vi "EdgeDetection_Setting_UI.vi"(6 "Analysis_Setting IN":T2={"PreProcess"=enum."*Algorithm*", "Parameter"=""}, 8 "error in (no error)":errorcluster, 9 "ProjectName":string, 10 "ROI List IN":refnum<vi>, 11 "Vision_Image":T8(plugin-control)) -> (0 "error out":errorcluster, 1 "Cancel?":bool, 3 "Analysis_Setting":T2={"PreProcess"=enum."*Algorithm*", "Parameter"=""})   [LabVIEW 2019]
uses:
  <vilib>/userdefined/High Color/IMAQdx.ctl
  <vilib>/vision/NI_Vision_Development_Module.lvlib
  Controls/_UI Command Cluster/Edge Detection_UI Command Cluster.ctl
  Controls/Edge Detection/Analysis_Edge Detection_Parameter.ctl
  Controls/Analysis_Type.ctl
  Controls/Analysis_Setting.ctl
  Controls/V_Analysis_Type.ctl
  <vilib>/vision/Measure.llb/Edge New.ctl
  Ctrl/VisionProcessName.ctl
panel:
  in  "Snap?":bool
  in  "ROI Descriptor":T1
  out "Numeric":i32
  in  "Done":bool
  in  "Cancel":bool
  in  "EdgeDetectionTab":T4(tab)
  in  "Number of Matches Requested":i32=1 min=1 max=9999
  in  "Process":T5(ring)=enum."Get All Edges"
  in  "Edge Options":T6={"Edge Polarity"=enum."All Edges", "Kernel Size"=3, "Width"=5, "Minimum Edge Strength"=10.0, "Interpolation Type"=enum."Bilinear", "Data Processing Method"=enum."Average"} {"Width" min=1 step=2; "Kernel Size" min=3 step=2; "Minimum Edge Strength" min=0.0 max=255.0 format="%.2g"}
  out "Number of Edges Detected":i32
  out "Edge Information":T7[](array[typedef]) {"Distance (Real-World)" format="%.2f"; "Location (Real-World)"."Y" format="%.2g"; "Location (Real-World)"."X" format="%.2f"; "Noise" format="%.2f"; "Location (Pixel)"."Y" format="%.2g"; "Location (Pixel)"."X" format="%.2f"; "Strength" format="%.2f"; "Distance (Pixel)" format="%.2f"}
  in  "Edge Detection_UI Command":T9(ring)
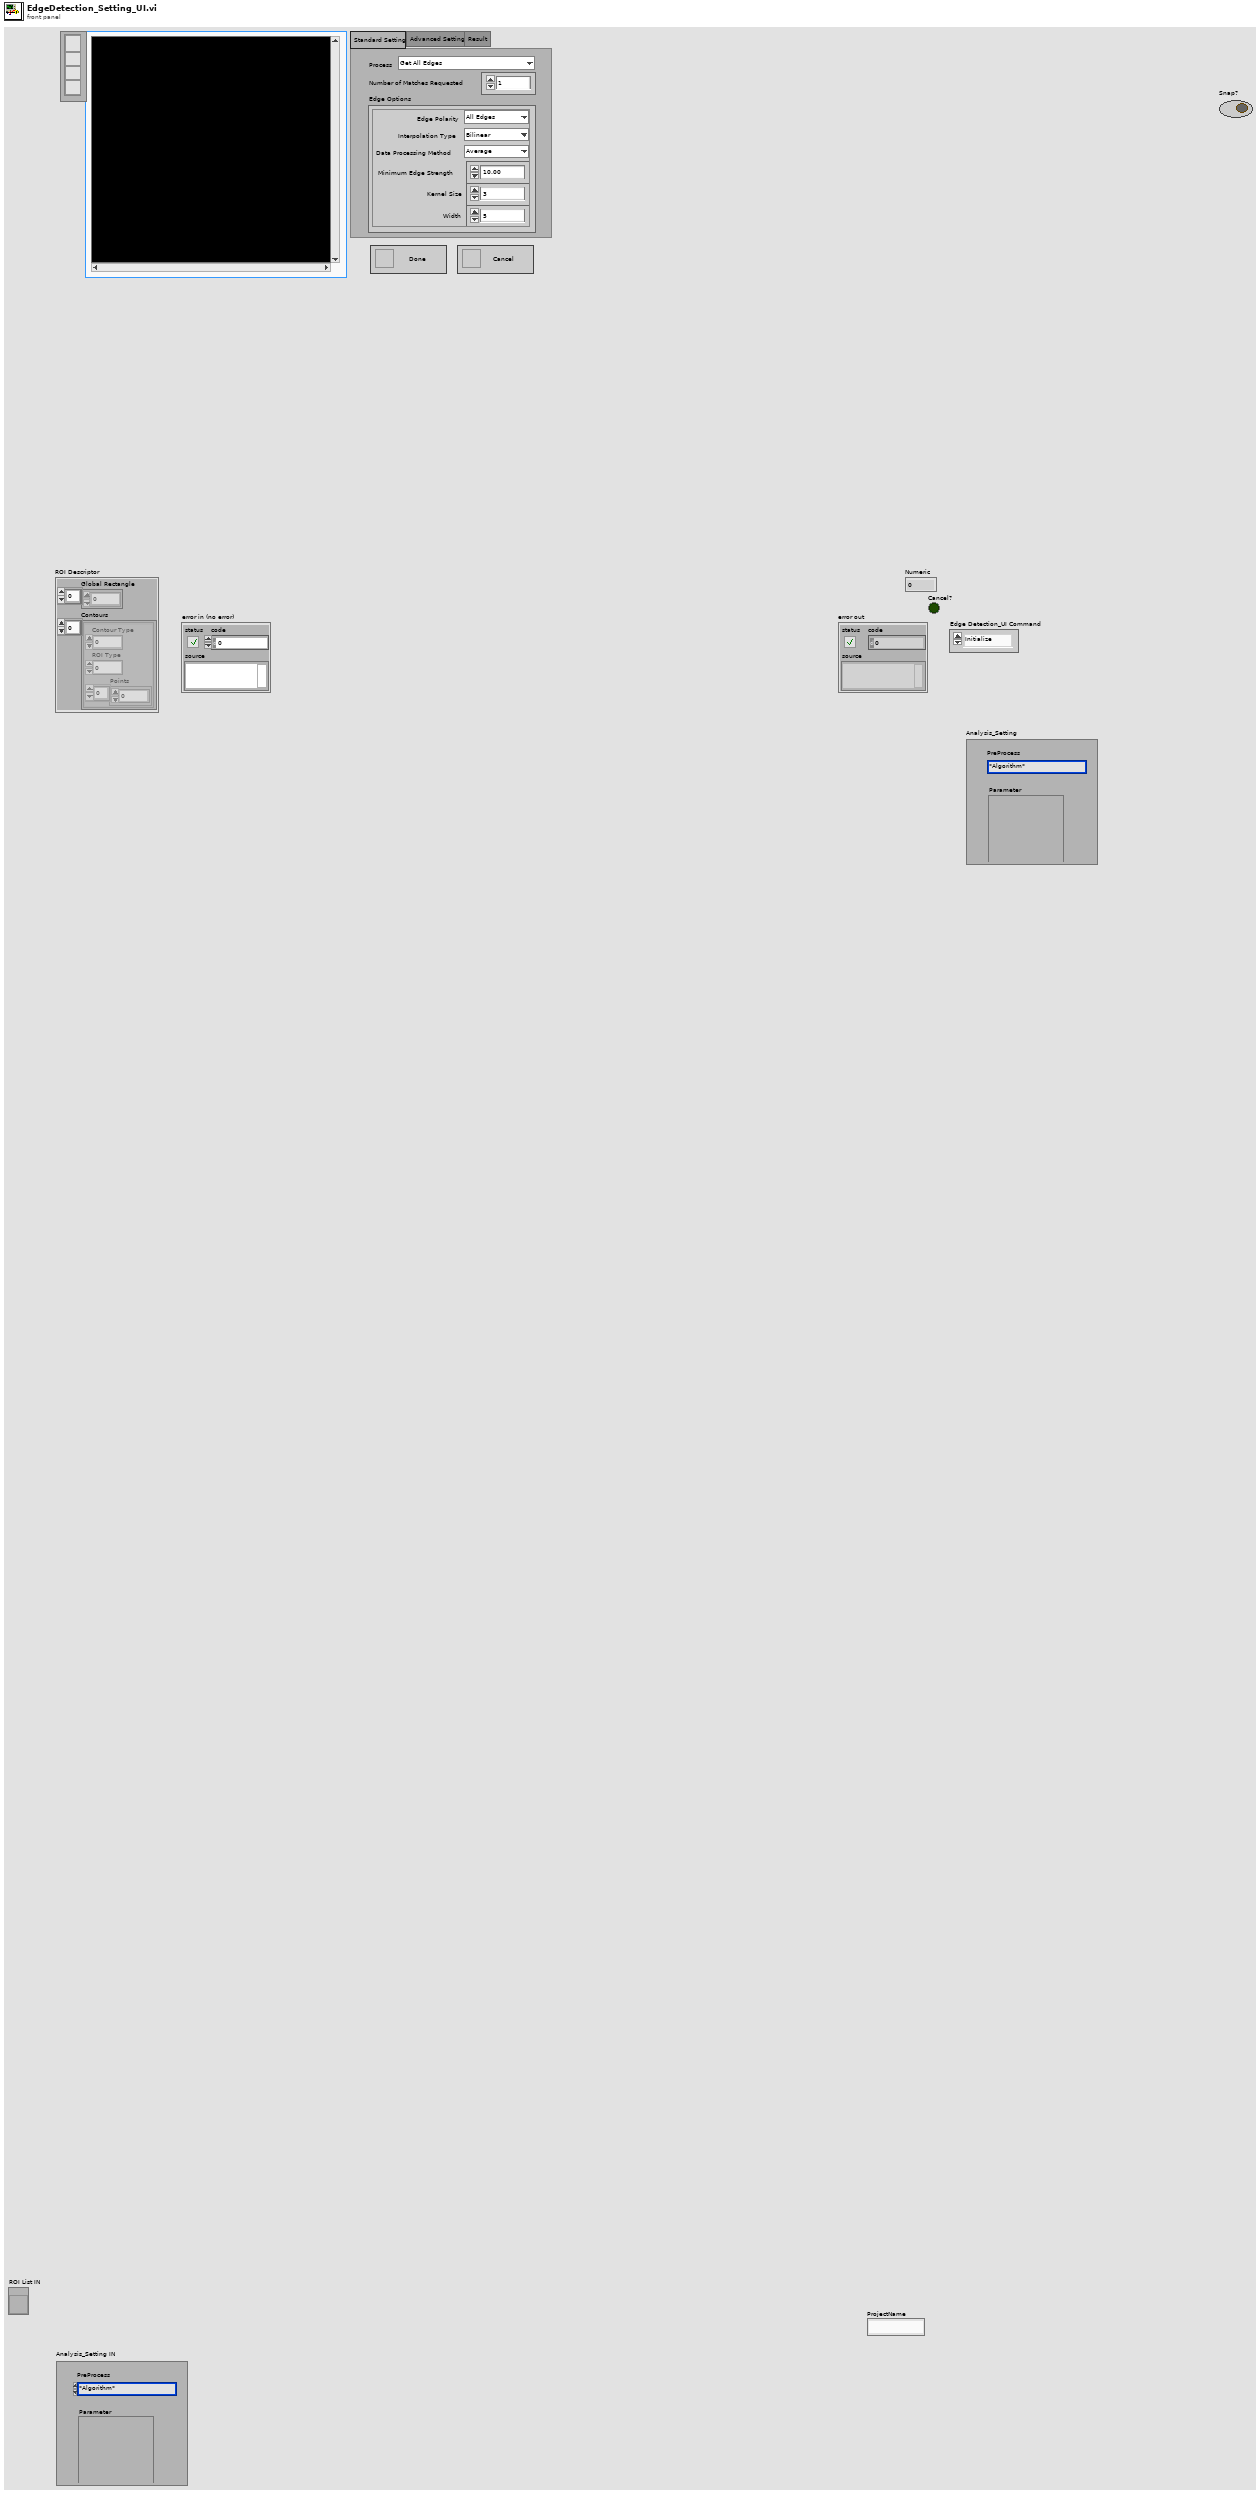
[diagram p1: front panel]
types:
  T1 = cluster{"Global Rectangle":i32[], "Contours":cluster{"Contour Type":u32, "ROI Type":u32, "Points":i32[]}[]}
  T2 = typedef "Analysis_Setting.ctl" = cluster{"PreProcess":T3, "Parameter":string}
  T3 = typedef "VisionProcessName.ctl" = enum16{"*CamParameter*", "CamAttributes", "*Preprocess*", "CG_Brightness", "C_Plane Extraction", "C_Threshold", "G_Lookup Table", "G_Threshold", "B_Image Inversion", "*Algorithm*", "CG_Histogram", "C_Color Matching", "C_Color Pattern Matching", "G_PatternMatch", "CG_Find Straight Edge", "CG_Adv. Find Straight Edge", "CG_Find Circular Edge", "G_Max Clamp", "G_Clamp (Rake)", "G_Pattern Matching"}
  T4 = enum32{"Standard Setting", "Advanced Setting", "Result"}
  T5 = enum16{"Get First Edge", "Get First + Last Edge", "Get All Edges", "Get Best Edge"}
  T6 = cluster{"Edge Polarity":enum16{"All Edges", "Rising Edges", "Falling Edges"}, "Kernel Size":u32, "Width":u32, "Minimum Edge Strength":dbl, "Interpolation Type":enum16{"Zero Order", "Bilinear", "Bilinear Fixed"}, "Data Processing Method":enum16{"Average", "Median"}}
  T7 = typedef "Edge New.ctl" = cluster{"Location (Pixel)":cluster{"X":sgl, "Y":sgl}, "Location (Real-World)":cluster{"X":sgl, "Y":sgl}, "Distance (Pixel)":dbl, "Distance (Real-World)":dbl, "Strength":dbl, "Noise":dbl, "Rising?":bool}
  T8 = typedef "IMAQ Image.ctl" = refnum<image>
  T9 = enum16{"Initialize", "Done", "Run Algorithm", "Cancel"}
  T10 = typedef "Analysis_Edge Detection_Parameter.ctl" = cluster{"Edge Options":cluster{"Edge Polarity":u16, "Kernel Size":u32, "Width":u32, "Minimum Edge Strength":dbl, "Interpolation Type":u16, "Data Processing Method":u16}, "Process":u16, "Number of Matches Requested":i32, "ROI Descriptor":cluster{"Global Rectangle":i32[], "Contours":cluster{"Contour Type":u32, "ROI Type":u32, "Points":i32[]}[]}}
  T11 = typedef "Edge Detection_UI Command Cluster.ctl" = cluster{"Edge Detection_UI Command":enum16{"Initialize", "Done", "Run Algorithm", "Cancel"}, "Edge Options":cluster{"Edge Polarity":u16, "Kernel Size":u32, "Width":u32, "Minimum Edge Strength":dbl, "Interpolation Type":u16, "Data Processing Method":u16}, "Process":u16, "Number of Matches Requested":i32, "ROI Descriptor":cluster{"Global Rectangle":i32[], "Contours":cluster{"Contour Type":u32, "ROI Type":u32, "Points":i32[]}[]}, "Snap Simulation Mouse Down":bool}
  T12 = typedef "IMAQ Line" = cluster{"Start X":i32, "Start Y":i32, "End X":i32, "End Y":i32}
  T13 = typedef "IMAQdx.ctl" = refnum<k21>
  T14 = cluster{"Contour Type":u32, "ROI Type":u32, "Points":i32[]}
  T15 = cluster{"Edge Polarity":u16, "Kernel Size":u32, "Width":u32, "Minimum Edge Strength":dbl, "Interpolation Type":u16, "Data Processing Method":u16}
  T16 = typedef "Image Type" = u32
  T17 = typedef "Analysis_Type.ctl" = u16
  T18 = typedef "ROI Descriptor" = cluster{"Global Rectangle":i32[], "Contours":cluster{"ID":enum32{"External", "Internal"}, "Type":u32, "Coordinates":i32[]}[]}
  T19 = typedef "Analysis_Setting.ctl" = cluster{"PreProcess":T20, "Parameter":string}
  T20 = typedef "V_Analysis_Type.ctl" = enum16{"None", "C_Color Pattern Matching", "G_PatternMatching", "G_ShapeDectect", "G_GeometricMatch", "B_Area Check"}
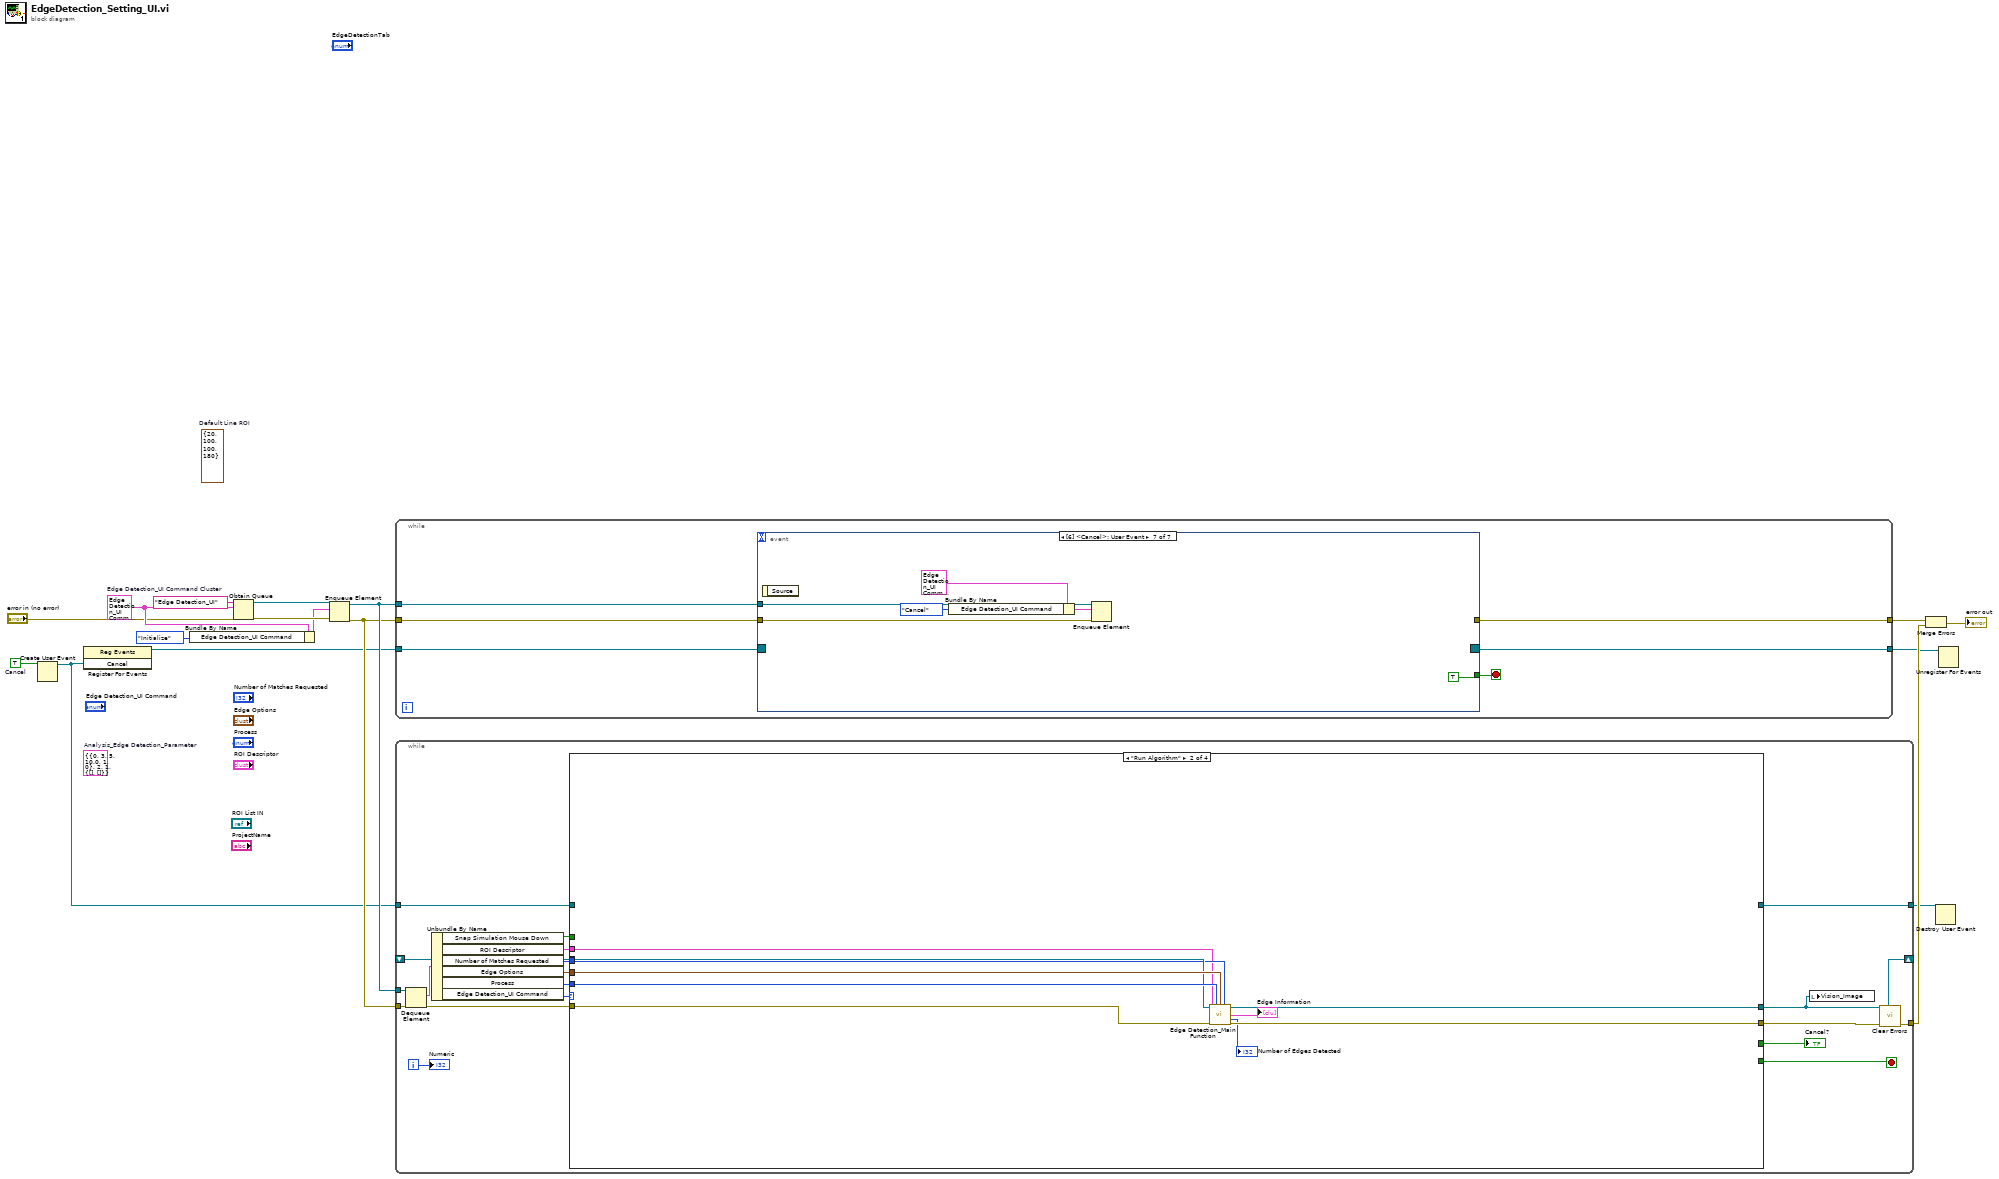
[diagram p0: block diagram]
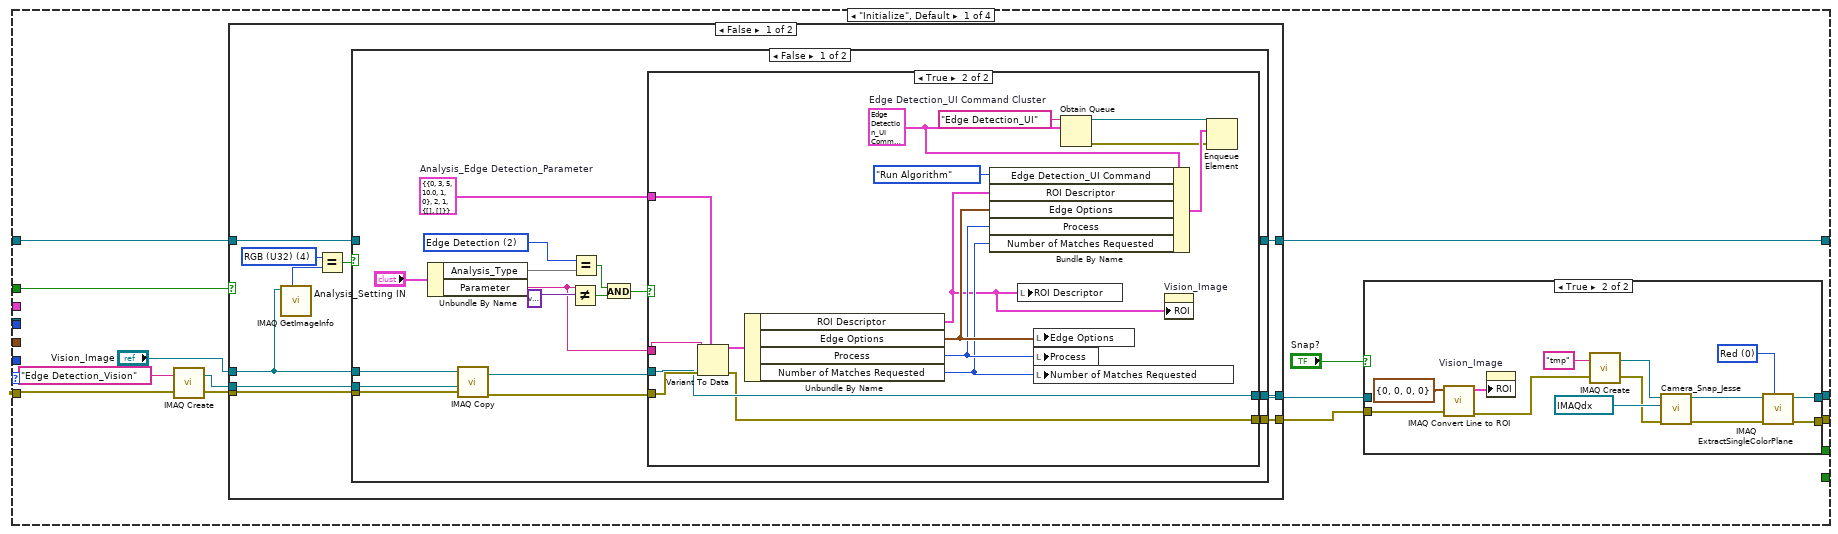
[diagram p2: hidden frame]
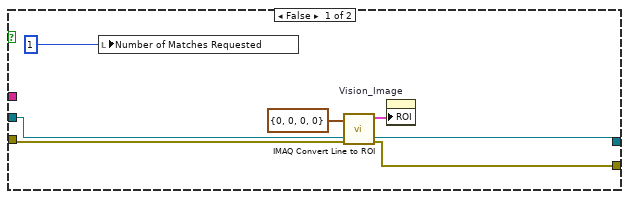
[diagram p4: hidden frame]
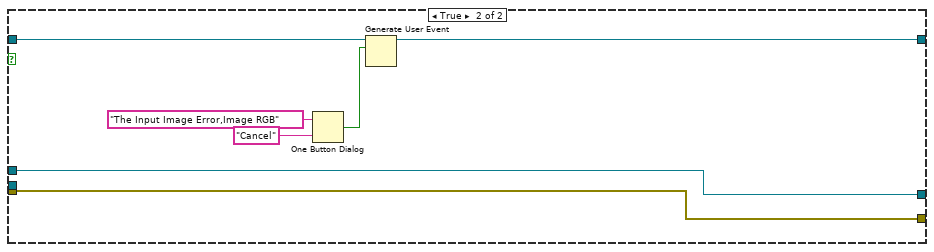
[diagram p5: hidden frame]
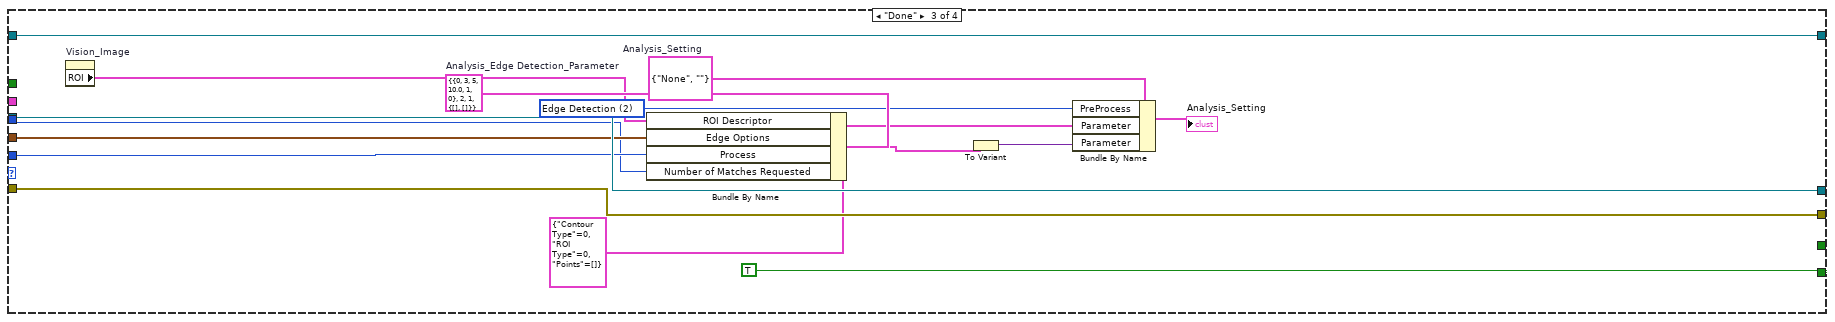
[diagram p7: hidden frame]
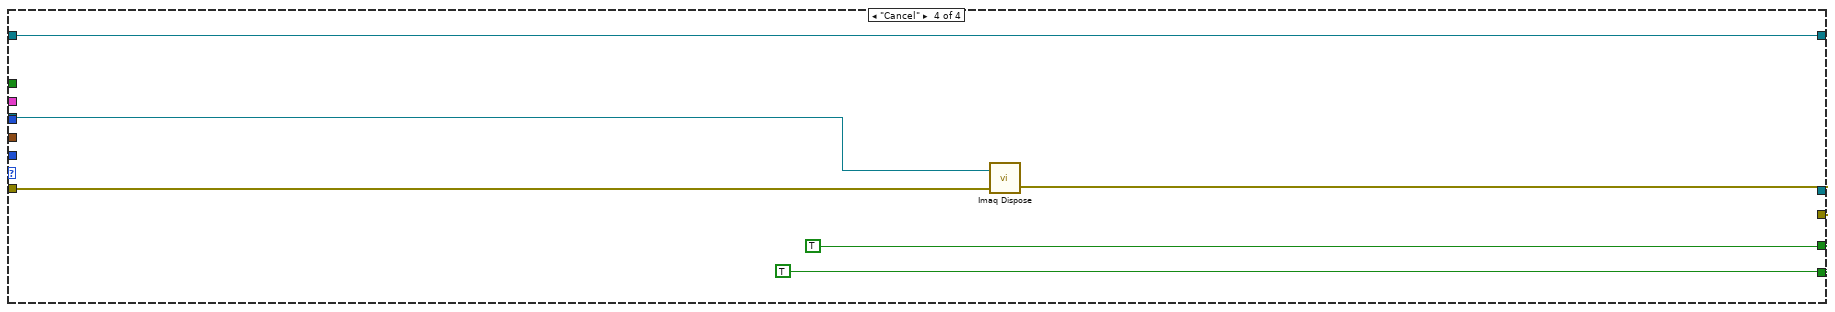
[diagram p8: hidden frame]
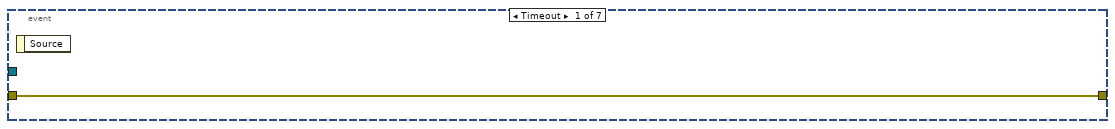
[diagram p9: hidden frame]
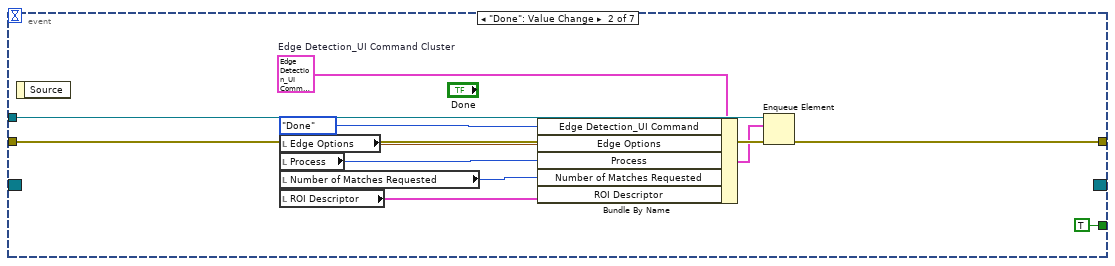
[diagram p10: hidden frame]
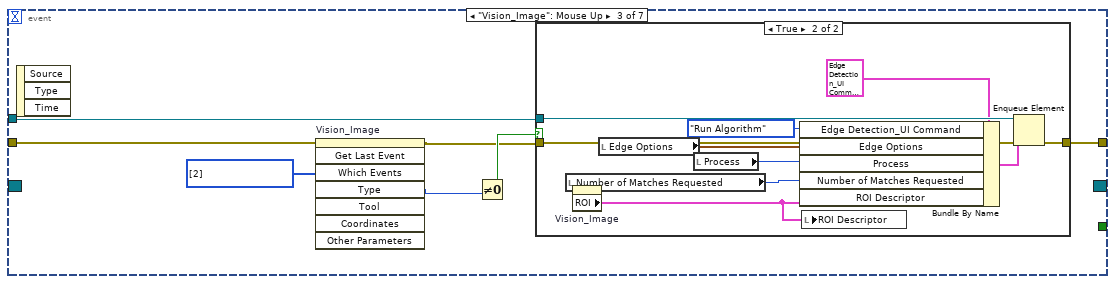
[diagram p11: hidden frame]
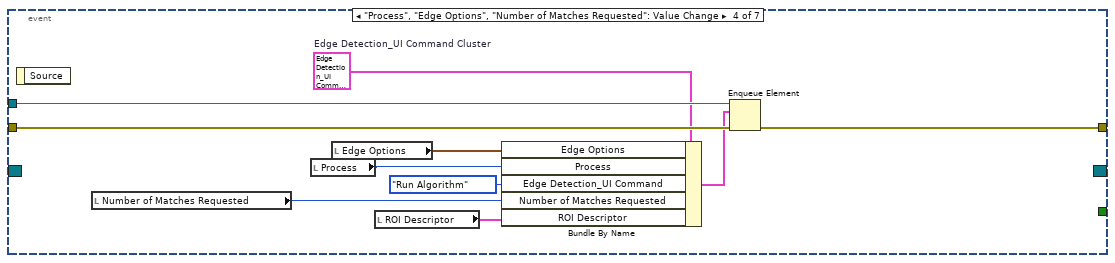
[diagram p13: hidden frame]
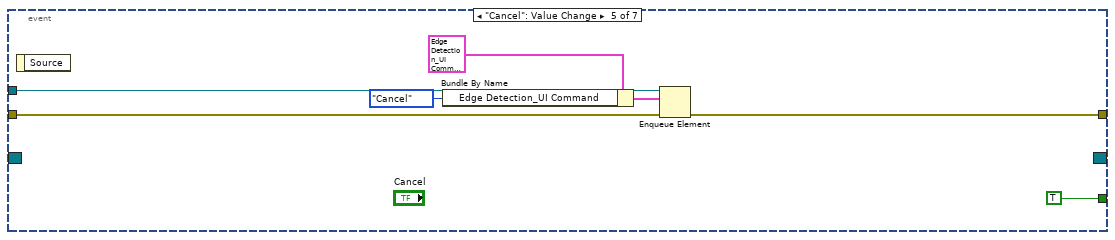
[diagram p14: hidden frame]
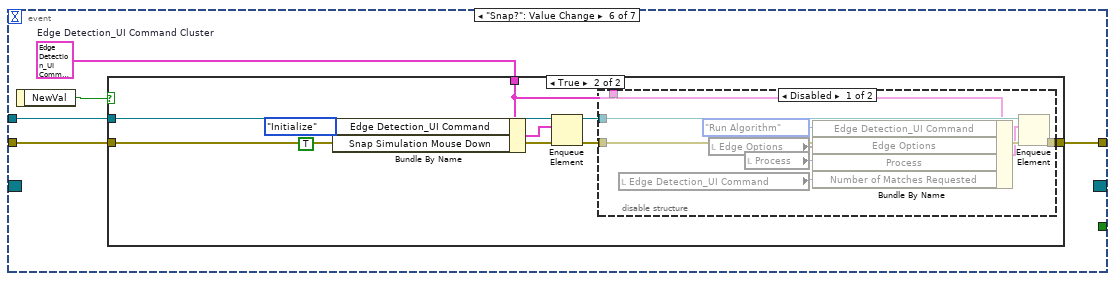
[diagram p15: hidden frame]
diagram:
  (unwired) T10 {"Edge Options"={"Edge Polarity"=0, "Kernel Size"=3, "Width"=5, "Minimum Edge Strength"=10.0, "Interpolation Type"=1, "Data Processing Method"=0}, "Process"=2, "Number of Matches Requested"=1, "ROI Descriptor"={"Global Rectangle"=[], "Contours"=[]}}  # Analysis_Edge Detection_Parameter
  w5 = TRUE  # Cancel
  w10 = T11 {"Edge Detection_UI Command"=enum."Initialize", "Edge Options"={"Edge Polarity"=0, "Kernel Size"=3, "Width"=5, "Minimum Edge Strength"=10.0, "Interpolation Type"=1, "Data Processing Method"=0}, "Process"=2, "Number of Matches Requested"=1, "ROI Descriptor"={"Global Rectangle"=[], "Contours"=[]}, "Snap Simulation Mouse Down"=FALSE}  # Edge Detection_UI Command Cluster
  (unwired) T12 {"Start X"=20, "Start Y"=100, "End X"=100, "End Y"=180}  # Default Line ROI
  n1 = Create User Event(user event datatype=w5) -> (user event=w3:refnum<user-event>)  [unwired: 1 in, 1 out]
  n2 = register-events(w3) -> (reference out=w4:refnum<event-registration>)  [unwired: 2 in, 1 out]
  n3 = Bundle By Name(cluster=w10, "Edge Detection_UI Command"=T9."Initialize") -> (w9:T11)
  n4 = Obtain Queue(name (unnamed)="Edge Detection_UI", element data type=w10, error in (no error)="error in (no error)") -> (queue out=w17:refnum<queue>, error out=w16:errorcluster)  [unwired: 2 in, 1 out]
  n5 = Enqueue Element(queue=w17, element=w9, error in (no error)=w16) -> (queue out=w14:refnum<queue>, error out=w13:errorcluster)  [unwired: 1 in, 1 out]
  n6 = while {
    tunnel: w14 -> [w36]
    tunnel: w13 -> [w35]
    shift-right: [w26] -> _
    shift-left: _ -> [w29]
    tunnel: [w19] -> w11
    tunnel: w3 -> [w21]
    tunnel: [w20] -> w1
    i -> [w27]
    stop <- w30 stop-if-true
    n7 = Dequeue Element(queue=w36, error in (no error)=w35) -> (element=w32:T11, error out=w33:errorcluster)  [unwired: 1 in, 2 out]
    n8 = Unbundle By Name(w32) -> ("Snap Simulation Mouse Down"=w22:bool, "ROI Descriptor"=w23:T1, "Number of Matches Requested"=w24:i32, "Edge Options"=w31:T15, "Process"=w28:u16, "Edge Detection_UI Command"=w34:T9)
    n9 = case shown="\"Run Algorithm\"" w34 {
      tunnel: w33 -> [w48 w131 w145 w150]
      tunnel: [w40 w128 w145 w149] -> w18
      tunnel: w31 -> [_ w130 w143 _]
      tunnel: [_ _ TRUE TRUE] -> w30
      tunnel: [w41 w127 w144 _] -> w26
      tunnel: w29 -> [_ w126 w144 w151]
      tunnel: w28 -> [_ w129 w142 _]
      tunnel: [_ _ _ TRUE] -> w25
      tunnel: w24 -> [_ w125 w134 _]
      tunnel: w23 -> [_ w123 _ _]
      tunnel: w22 -> [w47 _ _ _]
      tunnel: w21 -> [w38 _ w132 w147]
      tunnel: [w37 _ w132 w147] -> w20
      frame "Initialize", Default {
        n10 = call "IMAQ Create"("Image Name"="Edge Detection_Vision", "error in (no error)"=w48) -> ("New Image"=w46:T8, "error out"=w45:errorcluster)  [unwired: 3 in]
        n11 = case shown="False" w47 {
          tunnel: [w74 w120] -> w42
          tunnel: [w73 w121] -> w43
          tunnel: w45 -> [w72 w120]
          tunnel: "Vision_Image" -> [w70 _]
          tunnel: w46 -> [w71 w121]
          tunnel: w38 -> [w66 _]
          tunnel: [w65 _] -> w37
          frame False {
            w68 = T16 4 items=["Grayscale (U8)", "Grayscale (I16)", "Grayscale (SGL)", "Complex (CSG)", "RGB (U32)", "HSL (U32)", "RGB (U64)", "Grayscale (U16)"] ("x")
            n12 = call "IMAQ GetImageInfo"("Image"=w70) -> ("Image Type"=w69:T16)  [unwired: 3 in, 7 out]
            n13 = Equal?(x=w68, y=w69) -> (x = y?=w67:bool)
            n14 = case shown="False" w67 {
              tunnel: [w90 w117] -> w74
              tunnel: [w89 w114] -> w73
              tunnel: w72 -> [w79 w117]
              tunnel: w71 -> [w76 _]
              tunnel: w70 -> [w75 w114]
              tunnel: w66 -> [_ w115]
              tunnel: [_ w113] -> w65
              frame False {
                w80 = T10 {"Edge Options"={"Edge Polarity"=0, "Kernel Size"=3, "Width"=5, "Minimum Edge Strength"=10.0, "Interpolation Type"=1, "Data Processing Method"=0}, "Process"=2, "Number of Matches Requested"=1, "ROI Descriptor"={"Global Rectangle"=[], "Contours"=[]}}  # Analysis_Edge Detection_Parameter
                w86 = T17 2 items=["None", "PatternMatch", "Edge Detection", "Barcode 1D", "Barcode 2D", "Clamp", "Clamp MAX", "Particle", "Histogram", "Straight Edge", "Circle", "Shape Detect", "OCR", "Contour", "ColorMatch"] ("x")
                n15 = Unbundle By Name("Analysis_Setting IN") -> ("Analysis_Type"=w85, "Parameter"=w82:string)
                n16 = call "IMAQ Copy"("error in (no error)"=w79, "Image Dst"=w76, "Image Src"=w75) -> ("error out"=w77:errorcluster, "Image Dst Out"=w78:T8)  [unwired: 3 in]
                n17 = Not Equal?(x=w82, y=variant) -> (x != y?=w87:bool)
                n18 = Equal?(x=w86, y=w85) -> (x = y?=w88:bool)
                n19 = And(x=w88, y=w87) -> (x .and. y?=w83:bool)
                n20 = case shown="True" w83 {
                  tunnel: w77 -> [w92 w110]
                  tunnel: [w91 w98] -> w90
                  tunnel: [w95 w99] -> w89
                  tunnel: w82 -> [_ w112]
                  tunnel: w78 -> [w95 w99]
                  tunnel: w80 -> [_ w103]
                  frame False {
                    n21 = local write "Number of Matches Requested"(1 ("Number of Matches Requested")) -> ()
                    n22 = call "IMAQ Convert Line to ROI"("error in (no error)"=w92, "Line"=T12 {"Start X"=0, "Start Y"=0, "End X"=0, "End Y"=0}) -> ("error out"=w91:errorcluster, "ROI Descriptor"=w93:T18)  [unwired: 7 in]
                    n23 = property on="Vision_Image" class="ImageControl"("ROI"=w93) -> ()  [unwired: 2 in, 2 out]
                  }
                  frame True {
                    w108 = T11 {"Edge Detection_UI Command"=enum."Initialize", "Edge Options"={"Edge Polarity"=0, "Kernel Size"=3, "Width"=5, "Minimum Edge Strength"=10.0, "Interpolation Type"=1, "Data Processing Method"=0}, "Process"=2, "Number of Matches Requested"=1, "ROI Descriptor"={"Global Rectangle"=[], "Contours"=[]}, "Snap Simulation Mouse Down"=FALSE}  # Edge Detection_UI Command Cluster
                    n24 = Variant To Data(error in=w110, type=w103, Variant=w112) -> (data=w111:T10, error out=w98:errorcluster)
                    n25 = Unbundle By Name(w111) -> ("ROI Descriptor"=w97:T1, "Edge Options"=w102:T15, "Process"=w101:u16, "Number of Matches Requested"=w100:i32)
                    n26 = Bundle By Name(cluster=w108, "Edge Detection_UI Command"=T9."Run Algorithm", "ROI Descriptor"=w97, "Edge Options"=w102, "Process"=w101, "Number of Matches Requested"=w100) -> (w109:T11)
                    n27 = local write "ROI Descriptor"(w97) -> ()
                    n28 = local write "Edge Options"(w102) -> ()
                    n29 = local write "Process"(w101) -> ()
                    n30 = local write "Number of Matches Requested"(w100) -> ()
                    n31 = Obtain Queue(name (unnamed)="Edge Detection_UI", element data type=w108) -> (queue out=w105:refnum<queue>, error out=w106:errorcluster)  [unwired: 3 in, 1 out]
                    n32 = property on="Vision_Image" class="ImageControl"("ROI"=w97) -> ()  [unwired: 2 in, 2 out]
                    n33 = Enqueue Element(queue=w105, element=w109, error in (no error)=w106) -> ()  [unwired: 1 in, 3 out]
                  }
                }
              }
              frame True {
                n34 = One Button Dialog(message="The Input Image Error,Image RGB", button name ("OK")="Cancel") -> (true=w116:bool)
                n35 = Generate User Event(user event=w115, event data cluster=w116) -> (user event out=w113:refnum<user-event>)  [unwired: 2 in, 1 out]
              }
            }
          }
          frame True {
          }
        }
        n36 = case shown="True" "Snap?" {
          tunnel: [w51 w57] -> w40
          tunnel: [w50 w56] -> w41
          tunnel: w42 -> [w51 w53]
          tunnel: w43 -> [w50 _]
          frame False {
          }
          frame True {
            w60 = 0 items=["Red", "Green", "Blue", "Hue", "Saturation", "Luminance", "Value", "Intensity"] ("Color Plane")
            n37 = call "IMAQ Convert Line to ROI"("error in (no error)"=w53, "Line"=T12 {"Start X"=0, "Start Y"=0, "End X"=0, "End Y"=0}) -> ("error out"=w52:errorcluster, "ROI Descriptor"=w54:T18)  [unwired: 7 in]
            n38 = property on="Vision_Image" class="ImageControl"("ROI"=w54) -> ()  [unwired: 2 in, 2 out]
            n39 = call "IMAQ Create"("Image Name"="tmp", "error in (no error)"=w52) -> ("New Image"=w62:T8, "error out"=w59:errorcluster)  [unwired: 3 in]
            n40 = call "Camera_Snap_Jesse.vi"("error in (no error)"=w59, "Camera Session In"=T13 "cam0", "Image In"=w62) -> ("error out"=w58:errorcluster, "New Image"=w61:T8)  [unwired: 7 in]
            n41 = call "IMAQ ExtractSingleColorPlane"("Color Plane"=w60, "error in (no error)"=w58, "Image Src"=w61) -> ("error out"=w57:errorcluster, "Image Dst Out"=w56:T8)  [unwired: 1 in, 6 out]
          }
        }
      }
      frame "Run Algorithm" {
        n42 = call "Edge Detection_Main Function.vi"("Refnum in"=w126, "Process"=w129, "Edge Options"=w130, "Number of Matches Requested IN"=w125, "ROI"=w123, "error in (no error)"=w131) -> ("Image Out"=w127:T8, "Edge Information"=→"Edge Information":T7[], "Number of Edges Detected"=→"Number of Edges Detected":i32, "error out"=w128:errorcluster)  [unwired: 6 in]
      }
      frame "Done" {
        w139 = T17 2 items=["None", "PatternMatch", "Edge Detection", "Barcode 1D", "Barcode 2D", "Clamp", "Clamp MAX", "Particle", "Histogram", "Straight Edge", "Circle", "Shape Detect", "OCR", "Contour", "ColorMatch"] ("Analysis_Type")
        w141 = T10 {"Edge Options"={"Edge Polarity"=0, "Kernel Size"=3, "Width"=5, "Minimum Edge Strength"=10.0, "Interpolation Type"=1, "Data Processing Method"=0}, "Process"=2, "Number of Matches Requested"=1, "ROI Descriptor"={"Global Rectangle"=[], "Contours"=[]}}  # Analysis_Edge Detection_Parameter
        w140 = T19 {"PreProcess"=enum."None", "Parameter"=""}  # Analysis_Setting
        n43 = property on="Vision_Image" class="ImageControl"() -> ("ROI"=w133:T1)  [unwired: 2 in, 2 out]
        n44 = Bundle By Name(cluster=w141, "ROI Descriptor"=w133, "Edge Options"=w143, "Process"=w142, "Number of Matches Requested"=w134) -> (w137:T10)
        n45 = To Variant(anything=w137) -> (Variant=w136:variant)
        n46 = Bundle By Name(cluster=w140, "PreProcess"=w139, "Parameter"=T14 {"Contour Type"=0, "ROI Type"=0, "Points"=[]} ("RegionContour"), "Parameter"=w136) -> (→"Analysis_Setting":T19)
      }
      frame "Cancel" {
        n47 = call "Imaq Dispose"("Image"=w151, "error in (no error)"=w150) -> ("error out"=w149:errorcluster)  [unwired: 4 in]
      }
    }
    "Cancel?" <- w25
    n48 = local write "Vision_Image"(w26) -> ()
    n49 = call <vilib>:"Clear Errors.vi"("error in (no error)"=w18) -> ("error out"=w19:errorcluster)  [unwired: 5 in, 1 out]
    "Numeric" <- w27
  }
  n50 = while {
    tunnel: w14 -> [w158]
    tunnel: w13 -> [w157]
    tunnel: [w155] -> w12
    tunnel: w4 -> [w154]
    tunnel: [w153] -> w2
    stop <- w156 stop-if-true
    n51 = event shown="[6] <Cancel>: User Event" {
      selector: w154 -> [_ _ _ _ _ _ _]
      dyn-events: [_ _ _ _ _ _ _] -> w153
      timeout: _ -> [_ _ _ _ _ _ _]
      tunnel: w158 -> [_ w170 w177 w198 w205 w209 w232]
      tunnel: w157 -> [w159 w169 w174 w197 w204 w208 w231]
      tunnel: [_ TRUE _ _ TRUE _ TRUE] -> w156
      tunnel: [w159 w166 w171 w194 w199 w207 _] -> w155
      event Timeout {
        n52 = event-data() -> ()  [unwired: 1 in, 1 out]
      }
      event "Done": Value Change {
        w164 = T11 {"Edge Detection_UI Command"=enum."Initialize", "Edge Options"={"Edge Polarity"=0, "Kernel Size"=3, "Width"=5, "Minimum Edge Strength"=10.0, "Interpolation Type"=1, "Data Processing Method"=0}, "Process"=2, "Number of Matches Requested"=1, "ROI Descriptor"={"Global Rectangle"=[], "Contours"=[]}, "Snap Simulation Mouse Down"=FALSE}  # Edge Detection_UI Command Cluster
        n53 = event-data() -> ()  [unwired: 1 in, 1 out]
        n54 = local read "Edge Options"() -> (w163:T6)
        n55 = local read "Process"() -> (w162:T5)
        n56 = local read "Number of Matches Requested"() -> (w161:i32)
        n57 = local read "ROI Descriptor"() -> (w160:T1)
        n58 = Bundle By Name(cluster=w164, "Edge Detection_UI Command"=T9."Done", "Edge Options"=w163, "Process"=w162, "Number of Matches Requested"=w161, "ROI Descriptor"=w160) -> (w167:T11)
        n59 = Enqueue Element(queue=w170, element=w167, error in (no error)=w169) -> (error out=w166:errorcluster)  [unwired: 1 in, 2 out]
      }
      event "Vision_Image": Mouse Up {
        w175 = i32[] [2] items=["No Event"=0, "Click Event"=1, "Draw Event"=2, "Size Event"=4, "Scroll Event"=5, "Double Click Event"=8] ("Which Events")
        n60 = event-data() -> ()  [unwired: 1 in, 3 out]
        n61 = invoke on="Vision_Image" class="ImageControl" method="Get Last Event"(error in=w174, "Which Events"=w175) -> (error out=w173:errorcluster, "Type"=w172:i32)  [unwired: 6 in, 6 out]
        n62 = Not Equal To 0?(x=w172) -> (x != 0?=w176:bool)
        n63 = case shown="True" w176 {
          tunnel: w177 -> [_ w188]
          tunnel: w173 -> [w178 w187]
          tunnel: [w178 w183] -> w171
          frame False {
          }
          frame True {
            n64 = local read "Number of Matches Requested"() -> (w180:i32)
            n65 = property on="Vision_Image" class="ImageControl"() -> ("ROI"=w179:T1)  [unwired: 2 in, 2 out]
            n66 = local read "Edge Options"() -> (w182:T6)
            n67 = local read "Process"() -> (w181:T5)
            n68 = Bundle By Name(cluster=T11 {"Edge Detection_UI Command"=enum."Run Algorithm", "Edge Options"={"Edge Polarity"=0, "Kernel Size"=3, "Width"=5, "Minimum Edge Strength"=10.0, "Interpolation Type"=1, "Data Processing Method"=0}, "Process"=2, "Number of Matches Requested"=1, "ROI Descriptor"={"Global Rectangle"=[], "Contours"=[]}, "Snap Simulation Mouse Down"=FALSE} ("element"), "Edge Detection_UI Command"=T9."Run Algorithm", "Edge Options"=w182, "Process"=w181, "Number of Matches Requested"=w180, "ROI Descriptor"=w179) -> (w185:T11)
            n69 = local write "ROI Descriptor"(w179) -> ()
            n70 = Enqueue Element(queue=w188, element=w185, error in (no error)=w187) -> (error out=w183:errorcluster)  [unwired: 1 in, 2 out]
          }
        }
      }
      event "Process", "Edge Options", "Number of Matches Requested": Value Change {
        w190 = T11 {"Edge Detection_UI Command"=enum."Initialize", "Edge Options"={"Edge Polarity"=0, "Kernel Size"=3, "Width"=5, "Minimum Edge Strength"=10.0, "Interpolation Type"=1, "Data Processing Method"=0}, "Process"=2, "Number of Matches Requested"=1, "ROI Descriptor"={"Global Rectangle"=[], "Contours"=[]}, "Snap Simulation Mouse Down"=FALSE}  # Edge Detection_UI Command Cluster
        n71 = event-data() -> ()  [unwired: 1 in, 1 out]
        n72 = local read "Number of Matches Requested"() -> (w193:i32)
        n73 = local read "Process"() -> (w192:T5)
        n74 = local read "Edge Options"() -> (w191:T6)
        n75 = local read "ROI Descriptor"() -> (w189:T1)
        n76 = Bundle By Name(cluster=w190, "Edge Options"=w191, "Process"=w192, "Edge Detection_UI Command"=T9."Run Algorithm", "Number of Matches Requested"=w193, "ROI Descriptor"=w189) -> (w195:T11)
        n77 = Enqueue Element(queue=w198, element=w195, error in (no error)=w197) -> (error out=w194:errorcluster)  [unwired: 1 in, 2 out]
      }
      event "Cancel": Value Change {
        n78 = event-data() -> ()  [unwired: 1 in, 1 out]
        n79 = Bundle By Name(cluster=T11 {"Edge Detection_UI Command"=enum."Initialize", "Edge Options"={"Edge Polarity"=0, "Kernel Size"=3, "Width"=5, "Minimum Edge Strength"=10.0, "Interpolation Type"=1, "Data Processing Method"=0}, "Process"=2, "Number of Matches Requested"=1, "ROI Descriptor"={"Global Rectangle"=[], "Contours"=[]}, "Snap Simulation Mouse Down"=FALSE} ("element"), "Edge Detection_UI Command"=T9."Cancel") -> (w201:T11)
        n80 = Enqueue Element(queue=w205, element=w201, error in (no error)=w204) -> (error out=w199:errorcluster)  [unwired: 1 in, 2 out]
      }
      event "Snap?": Value Change {
        w206 = T11 {"Edge Detection_UI Command"=enum."Initialize", "Edge Options"={"Edge Polarity"=0, "Kernel Size"=3, "Width"=5, "Minimum Edge Strength"=10.0, "Interpolation Type"=1, "Data Processing Method"=0}, "Process"=2, "Number of Matches Requested"=1, "ROI Descriptor"={"Global Rectangle"=[], "Contours"=[]}, "Snap Simulation Mouse Down"=FALSE}  # Edge Detection_UI Command Cluster
        n81 = event-data() -> ("NewVal"=w210:bool)  [unwired: 1 in]
        n82 = case shown="True" w210 {
          tunnel: w209 -> [_ w220]
          tunnel: w208 -> [w211 w219]
          tunnel: [w211 w215] -> w207
          tunnel: w206 -> [_ w213]
          frame False {
          }
          frame True {
            n83 = Bundle By Name(cluster=w213, "Edge Detection_UI Command"=T9."Initialize", "Snap Simulation Mouse Down"=TRUE) -> (w218:T11)
            n84 = Enqueue Element(queue=w220, element=w218, error in (no error)=w219) -> (queue out=w214:refnum<queue>, error out=w216:errorcluster)  [unwired: 1 in, 1 out]
            n85 = disable-structure shown="Disabled" {
              disable-tunnel: w216 -> [w229 _]
              disable-tunnel: [w228 _] -> w215
              disable-tunnel: w214 -> [w227 _]
              disable-tunnel: w213 -> [w226 _]
              frame Disabled {
                n86 = local read "Edge Detection_UI Command"() -> (w221:T9)
                n87 = local read "Edge Options"() -> (w224:T6)
                n88 = local read "Process"() -> (w223:T5)
                n89 = Bundle By Name(cluster=w226, "Edge Detection_UI Command"=T9."Run Algorithm", "Edge Options"=w224, "Process"=w223, "Number of Matches Requested"=w221) -> (w222:T11)
                n90 = Enqueue Element(queue=w227, element=w222, error in (no error)=w229) -> (error out=w228:errorcluster)  [unwired: 1 in, 2 out]
              }
              frame Enabled {
              }
            }
          }
        }
      }
      event User Event {
        n91 = event-data() -> ()  [unwired: 1 in, 1 out]
        n92 = Bundle By Name(cluster=T11 {"Edge Detection_UI Command"=enum."Initialize", "Edge Options"={"Edge Polarity"=0, "Kernel Size"=3, "Width"=5, "Minimum Edge Strength"=10.0, "Interpolation Type"=1, "Data Processing Method"=0}, "Process"=2, "Number of Matches Requested"=1, "ROI Descriptor"={"Global Rectangle"=[], "Contours"=[]}, "Snap Simulation Mouse Down"=FALSE} ("element"), "Edge Detection_UI Command"=T9."Cancel") -> (w233:T11)
        n93 = Enqueue Element(queue=w232, element=w233, error in (no error)=w231) -> ()  [unwired: 1 in, 3 out]
      }
    }
  }
  n94 = Merge Errors(w12, w11) -> (→"error out":errorcluster)
  n95 = Destroy User Event(user event=w1) -> ()  [unwired: 1 in, 1 out]
  n96 = Unregister For Events(event registration refnum=w2) -> ()  [unwired: 1 in, 1 out]
